vi "BallCollector.vi"(8 "error in\n(no error)":errorcluster) -> (0 "error out":errorcluster)   [LabVIEW 2017]
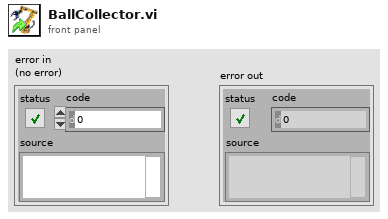
[diagram p1: front panel]
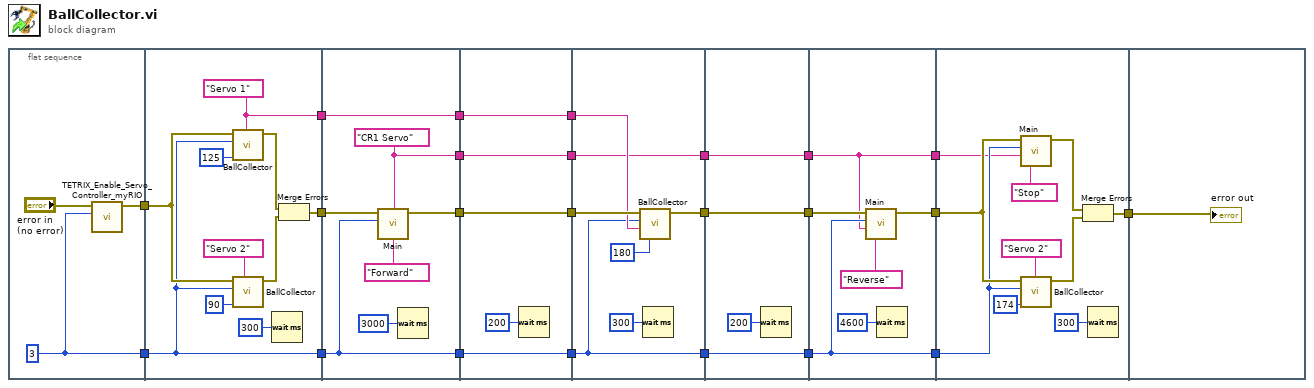
[diagram p0: block diagram]
diagram:
  n1 = flat-sequence {
    tunnel: [w26] -> w2
    tunnel: [w25] -> w1
    tunnel: w2 -> [w36]
    tunnel: w1 -> [w29]
    tunnel: [w30] -> w23
    tunnel: [w29] -> w22
    tunnel: [w28] -> w17
    tunnel: w23 -> [w43]
    tunnel: w22 -> [w39]
    tunnel: [w40] -> w20
    tunnel: [w39] -> w19
    tunnel: w17 -> [w38]
    tunnel: [w38] -> w16
    tunnel: [w37] -> w10
    tunnel: [w47] -> w21
    tunnel: w20 -> [w47]
    tunnel: w19 -> [w46]
    tunnel: [w46] -> w18
    tunnel: w16 -> [w45]
    tunnel: [w45] -> w15
    tunnel: w10 -> [w44]
    tunnel: [w44] -> w9
    tunnel: w21 -> [w55]
    tunnel: w18 -> [w51]
    tunnel: w15 -> [w54]
    tunnel: [w52] -> w13
    tunnel: [w51] -> w12
    tunnel: w9 -> [w50]
    tunnel: [w50] -> w8
    tunnel: [w58] -> w14
    tunnel: w13 -> [w58]
    tunnel: w12 -> [w57]
    tunnel: [w57] -> w11
    tunnel: w8 -> [w56]
    tunnel: [w56] -> w7
    tunnel: w14 -> [w65]
    tunnel: w11 -> [w61]
    tunnel: w7 -> [w60]
    tunnel: [w62] -> w6
    tunnel: [w61] -> w5
    tunnel: [w60] -> w4
    tunnel: w6 -> [w75]
    tunnel: w5 -> [w68]
    tunnel: w4 -> [w67]
    tunnel: [w69] -> w3
    tunnel: w3 -> [w76]
    frame #0 {
      w25 = u8 3 ("Controller ID#  (I2C Address)")
      n2 = call <vilib>:"TETRIX_Enable_Servo_Controller_myRIO.vi"("Controller ID#  (I2C Address)"=w25, "Error/Flow In"="error in\n(no error)") -> ("Error/Flow Out"=w26:errorcluster)  [unwired: 5 in]
    }
    frame #1 {
      w28 = "Servo 1" ("Select Channel")
      n3 = call "BallCollector.vi"("Set Servo Position (0 - 180 degrees)"=u8 125, "Select Channel"=w28, "Controller ID#  (I2C Address)"=w29, "Error/Flow In"=w36) -> ("Error/Flow Out"=w32:errorcluster)  [unwired: 3 in]
      n4 = call "BallCollector.vi"("Set Servo Position (0 - 180 degrees)"=u8 90, "Select Channel"="Servo 2", "Controller ID#  (I2C Address)"=w29, "Error/Flow In"=w36) -> ("Error/Flow Out"=w31:errorcluster)  [unwired: 3 in]
      n5 = Wait (ms)(milliseconds to wait=u32 300) -> ()  [unwired: 1 out]
      n6 = Merge Errors(w32, w31) -> (w30:errorcluster)
    }
    frame #2 {
      w37 = "CR1 Servo" ("Select Channel")
      n7 = call "Main.vi"("CR Servo State"="Forward", "Select Channel"=w37, "Controller ID#  (I2C Address)"=w39, "Error/Flow In"=w43) -> ("Error/Flow Out"=w40:errorcluster)  [unwired: 3 in]
      n8 = Wait (ms)(milliseconds to wait=u32 3000) -> ()  [unwired: 1 out]
    }
    frame #3 {
      n9 = Wait (ms)(milliseconds to wait=u32 200) -> ()  [unwired: 1 out]
    }
    frame #4 {
      n10 = call "BallCollector.vi"("Set Servo Position (0 - 180 degrees)"=u8 180, "Select Channel"=w54, "Controller ID#  (I2C Address)"=w51, "Error/Flow In"=w55) -> ("Error/Flow Out"=w52:errorcluster)  [unwired: 3 in]
      n11 = Wait (ms)(milliseconds to wait=u32 300) -> ()  [unwired: 1 out]
    }
    frame #5 {
      n12 = Wait (ms)(milliseconds to wait=u32 200) -> ()  [unwired: 1 out]
    }
    frame #6 {
      n13 = call "Main.vi"("CR Servo State"="Reverse", "Select Channel"=w60, "Controller ID#  (I2C Address)"=w61, "Error/Flow In"=w65) -> ("Error/Flow Out"=w62:errorcluster)  [unwired: 3 in]
      n14 = Wait (ms)(milliseconds to wait=u32 4600) -> ()  [unwired: 1 out]
    }
    frame #7 {
      n15 = call "Main.vi"("CR Servo State"="Stop", "Select Channel"=w67, "Controller ID#  (I2C Address)"=w68, "Error/Flow In"=w75) -> ("Error/Flow Out"=w71:errorcluster)  [unwired: 3 in]
      n16 = call "BallCollector.vi"("Set Servo Position (0 - 180 degrees)"=u8 174, "Select Channel"="Servo 2", "Controller ID#  (I2C Address)"=w68, "Error/Flow In"=w75) -> ("Error/Flow Out"=w70:errorcluster)  [unwired: 3 in]
      n17 = Merge Errors(w71, w70) -> (w69:errorcluster)
      n18 = Wait (ms)(milliseconds to wait=u32 300) -> ()  [unwired: 1 out]
    }
    frame #8 {
      "error out" <- w76
    }
  }
